vi "Drawing Epicycles.vi"() -> ()   [LabVIEW 2020]
panel:
  in  "Period":dbl
  in  "Number of Terms":dbl
  out "Time":dbl
  out "XY Graph":cluster{dbl[], dbl[]}[](graph)
  in  "Draw Circle?":bool
  in  "stop":bool
  in  "Done":bool
  in  "Pen Style":T1={"Width"=1, "Style"=enum."Solid"}
  out "Picture":picture
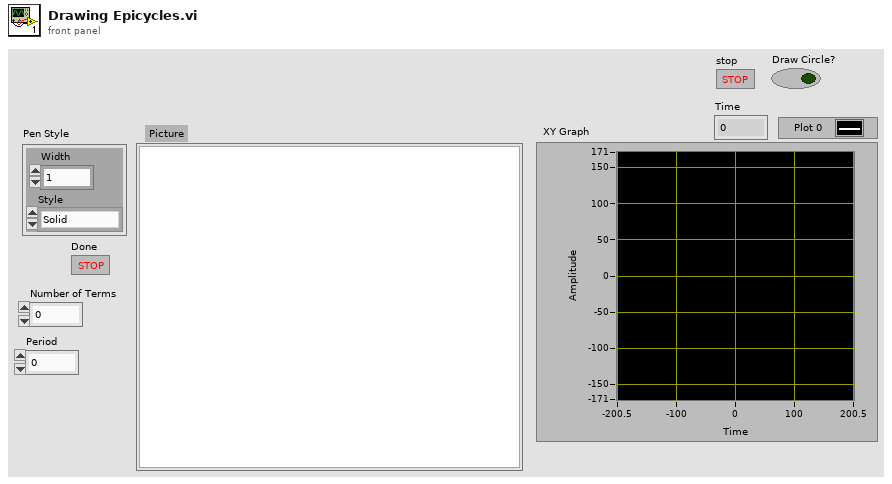
[diagram p1: front panel]
types:
  T1 = cluster{"Width":u16, "Style":enum32{"Solid", "Dash", "Dot", "DashDot", "DashDotDot"}}
  T2 = typedef "LVBoundsTypeDef.ctl" = cluster{"Width":u32, "Height":u32}
  T3 = typedef "LVMouseTypeDef.ctl" = cluster{"Mouse Position":cluster{"X":i32, "Y":i32}, "Mouse Modifiers":cluster{"Button Down":bool, "Shift Mod":bool, "Menu Mod":bool, "Option Mod":bool}}
  T4 = typedef "Component.ctl" = cluster{"Radius Formula":string, "Frequency":dbl, "Phase Offset":dbl}
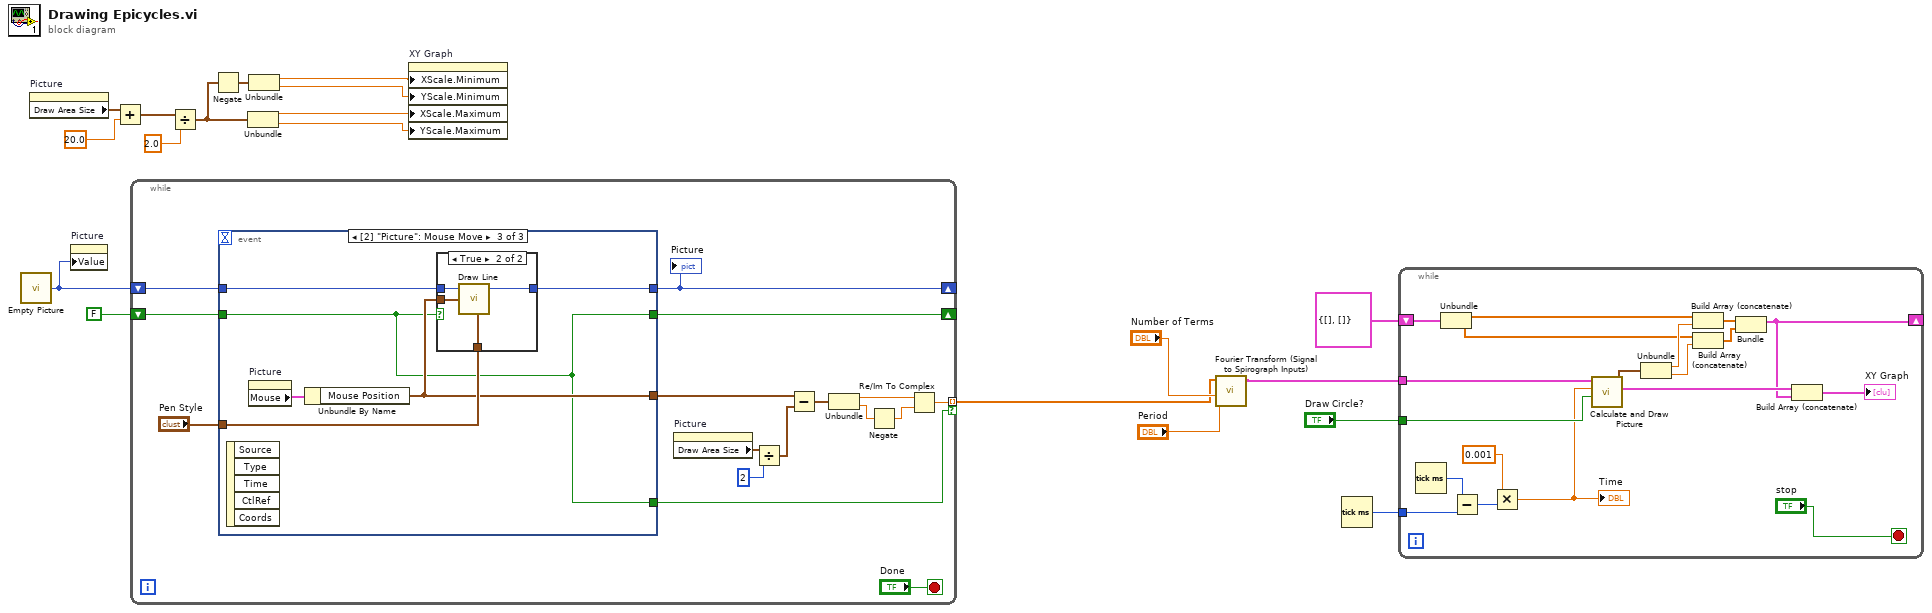
[diagram p0: block diagram]
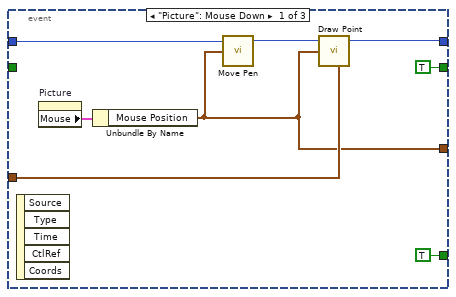
[diagram p2: hidden frame]
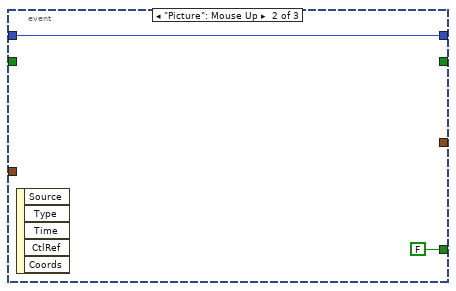
[diagram p3: hidden frame]
diagram:
  n1 = call "Empty Picture"() -> ("empty picture"=w18:picture)
  n2 = property on="Picture" class="Pict"() -> ("Draw Area Size"=w14:T2)  [unwired: 2 in, 2 out]
  n3 = property on="Picture" class="Pict"("Value"=w18) -> ()  [unwired: 2 in, 2 out]
  n4 = Add(x=w14, y=20.0) -> (x+y=w12:cluster{"Width":dbl, "Height":dbl})
  n5 = while {
    shift-right: [w34] -> _
    shift-left: w18 -> [w35]
    shift-right: [w32] -> _
    shift-left: FALSE -> [w33]
    tunnel: [w29] -> w1 mode=indexing if=w23
    stop <- "Done" stop-if-true
    n6 = event shown="[2] \"Picture\": Mouse Move" {
      selector: _ -> [_ _ _]
      dyn-events: _ -> [_ _ _]
      timeout: _ -> [_ _ _]
      tunnel: w35 -> [w43 w45 w51]
      tunnel: [w40 w45 w50] -> w34
      tunnel: w33 -> [_ _ w46]
      tunnel: [TRUE _ w46] -> w32
      tunnel: "Pen Style" -> [w38 _ w48]
      tunnel: [w37 _ w47] -> w26
      tunnel: [TRUE FALSE w46] -> w23
      event "Picture": Mouse Down {
        n7 = event-data() -> ()  [unwired: 1 in, 5 out]
        n8 = property on="Picture" class="Pict"() -> ("Mouse"=w41:T3)  [unwired: 2 in, 2 out]
        n9 = Unbundle By Name(w41) -> ("Mouse Position"=w37:cluster{"X":i32, "Y":i32})
        n10 = call <vilib>:"Move Pen.vi"("new position"=w37, "picture"=w43) -> ("new picture"=w42:picture)  [unwired: 3 in]
        n11 = call <vilib>:"Draw Point.vi"("picture"=w42, "point(x,y)"=w37, "pen"=w38) -> ("new picture"=w40:picture)  [unwired: 6 in]
      }
      event "Picture": Mouse Up {
        n12 = event-data() -> ()  [unwired: 1 in, 5 out]
      }
      event "Picture": Mouse Move {
        n13 = event-data() -> ()  [unwired: 1 in, 5 out]
        n14 = property on="Picture" class="Pict"() -> ("Mouse"=w49:T3)  [unwired: 2 in, 2 out]
        n15 = Unbundle By Name(w49) -> ("Mouse Position"=w47:cluster{"X":i32, "Y":i32})
        n16 = case shown="True" w46 {
          tunnel: w51 -> [w52 w56]
          tunnel: [w52 w55] -> w50
          tunnel: w47 -> [_ w54]
          tunnel: w48 -> [_ w53]
          frame False {
          }
          frame True {
            n17 = call <vilib>:"Draw Line.vi"("picture"=w56, "end point"=w54, "pen"=w53) -> ("new picture"=w55:picture)  [unwired: 6 in]
          }
        }
      }
    }
    "Picture" <- w34
    n18 = property on="Picture" class="Pict"() -> ("Draw Area Size"=w28:T2)  [unwired: 2 in, 2 out]
    n19 = Divide(x=w28, y=2 ("X")) -> (x/y=w25:cluster{"Width":dbl, "Height":dbl})
    n20 = Subtract(x=w26, y=w25) -> (x-y=w24:cluster{dbl, dbl})
    n21 = Unbundle(w24) -> (w30:dbl, w21:dbl)
    n22 = Negate(x=w21) -> (-x=w20:dbl)
    n23 = Re/Im To Complex(1:w20, 2:w30) -> (0:w29:cdb)
  }
  n24 = Divide(x=w12, y=2.0) -> (x/y=w16:cluster{"Width":dbl, "Height":dbl})
  n25 = Negate(x=w16) -> (-x=w15:cluster{"Width":dbl, "Height":dbl})
  n26 = Unbundle(w16) -> ("Width"=w9:dbl, "Height"=w8:dbl)
  n27 = Unbundle(w15) -> ("Width"=w11:dbl, "Height"=w10:dbl)
  n28 = property on="XY Graph" class="XYGraph (strict)"("XScale.Minimum"=w11, "YScale.Minimum"=w10, "XScale.Maximum"=w9, "YScale.Maximum"=w8) -> ()  [unwired: 2 in, 2 out]
  n29 = call "Fourier Transform (Signal to Spirograph Inputs).vi"("Number of Terms"="Number of Terms", "Period"="Period", "Signal"=w1) -> ("Inputs"=w5:T4[])  [unwired: 8 in]
  n30 = Tick Count (ms)() -> (millisecond timer value=w7:u32)
  n31 = while {
    tunnel: w5 -> [w72]
    tunnel: w7 -> [w75]
    tunnel: "Draw Circle?" -> [w73]
    shift-right: [w60] -> _
    shift-left: cluster{dbl[], dbl[]} {[], []} -> [w68]
    stop <- "stop" stop-if-true
    n32 = Tick Count (ms)() -> (millisecond timer value=w74:u32)
    n33 = Unbundle(w68) -> (w67:dbl[], w64:dbl[])
    n34 = Subtract(x=w74, y=w75) -> (x-y=w71:u32)
    n35 = Multiply(x=0.001, y=w71) -> (x*y=w59:dbl)
    "Time" <- w59
    n36 = call "Calculate and Draw Picture.vi"("Draw Circle?"=w73, "Time"=w59, "Inputs"=w72) -> ("Points"=w61:cluster{dbl[], dbl[]}[], "Endpoint"=w69:cluster{"x":dbl, "y":dbl})  [unwired: 7 in]
    n37 = Unbundle(w69) -> ("x"=w66:dbl, "y"=w65:dbl)
    n38 = Build Array (concatenate)(w67, w66) -> (w63:dbl[])
    n39 = Build Array (concatenate)(w64, w65) -> (w62:dbl[])
    n40 = Bundle(w63, w62) -> (w60:cluster{dbl[], dbl[]})  [unwired: 1 in]
    n41 = Build Array (concatenate)(w61, w60) -> (→"XY Graph":cluster{dbl[], dbl[]}[])
  }
